vi "email.vi"(1 "Body":string="[No Body]", 2 "Enable":bool) -> ()   [LabVIEW 2011]
panel:
  out "error out":errorcluster
  in  "CC (Carbon Copy Recipient - Optional)":string
  in  "Attachment - Optional":path
  in  "Port":i32=587
  in  "Enable SSL":bool=TRUE
  in  "GMAIL Account Password":string="joblhzitaafwukgr"
  in  "GMAIL Account User ID":string="hvac.labview"
  in  "Outgoing Mail Server (SMTP)":string="smtp.gmail.com"
  in  "Subject":string="Automatic Email: HVAC Project"
  in  "Recipient's Name":string="HVAC Member"
  in  "Recipient's Email":string="mani.amoozadeh2@gmail.com"
  in  "Sender's Name":string="hvac.labview"
  in  "Sender's Email":string="hvac.labview@gmail.com"
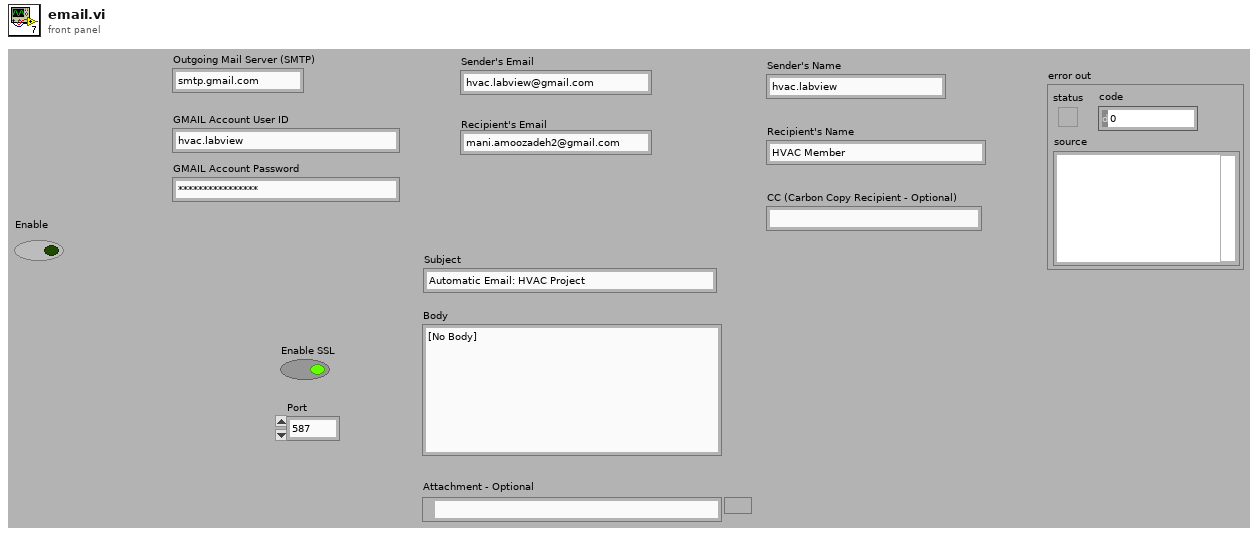
[diagram p1: front panel]
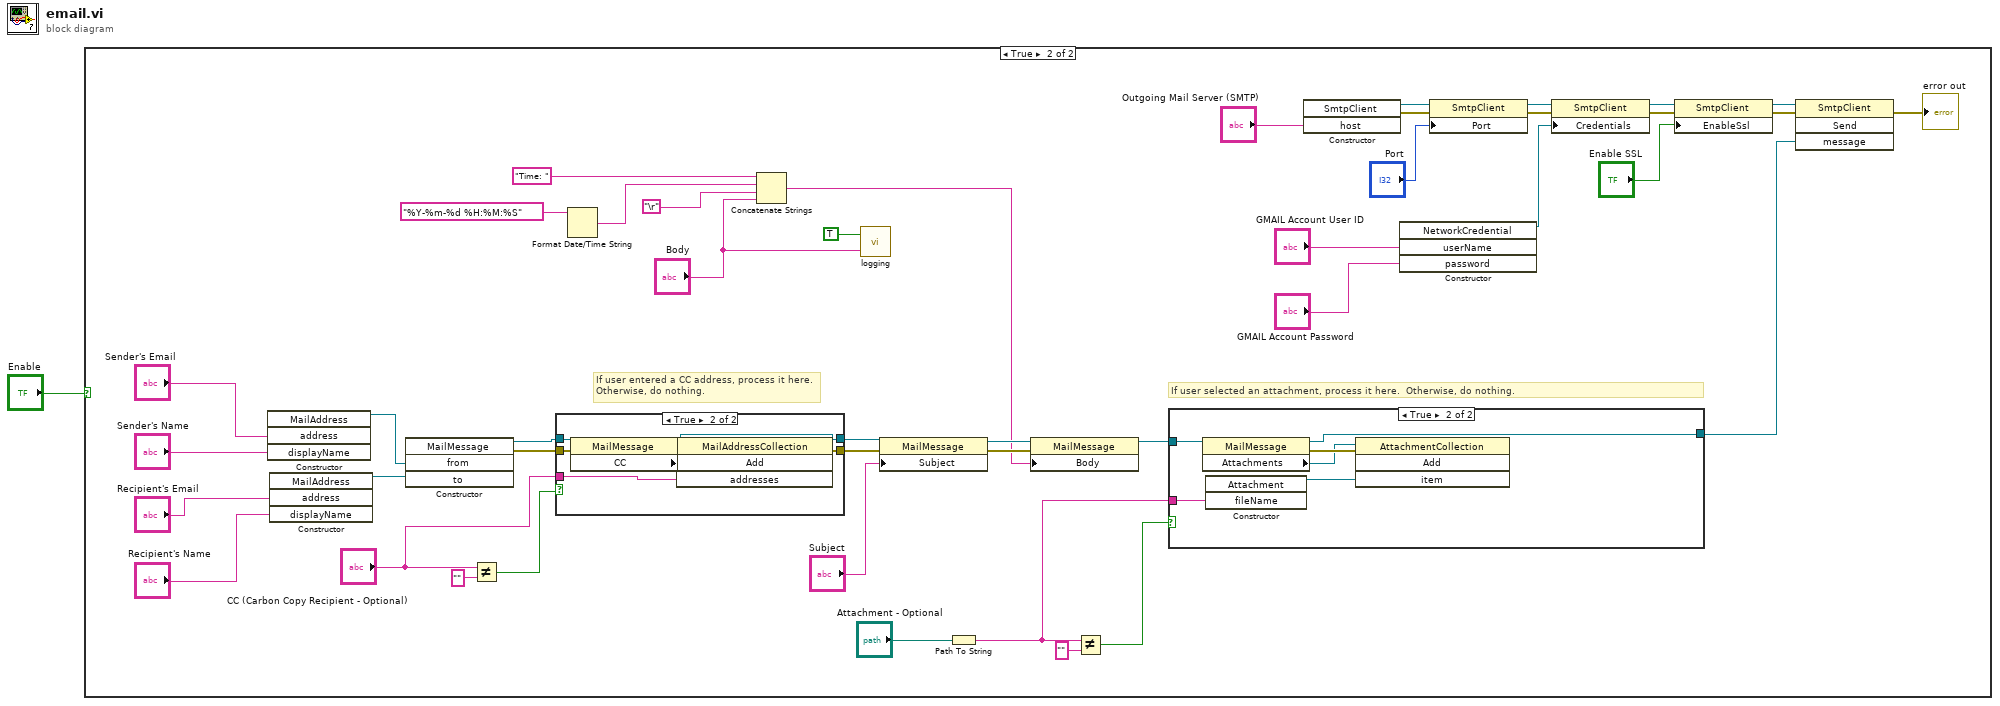
[diagram p0: block diagram]
diagram:
  n1 = case shown="True" "Enable" {
    frame False {
    }
    frame True {
      # "If user selected an attachment, process it here.  Otherwise, do nothing."
      # "If user entered a CC address, process it here.\nOtherwise, do nothing."
      n2 = constructor class="MailAddress"("address"="Sender's Email", "displayName"="Sender's Name") -> (reference out=w44:refnum<k24>)  [unwired: 3 in, 4 out]
      n3 = constructor class="MailAddress"("address"="Recipient's Email", "displayName"="Recipient's Name") -> (reference out=w45:refnum<k24>)  [unwired: 3 in, 4 out]
      n4 = constructor class="MailMessage"("from"=w44, "to"=w45) -> (reference out=w13:refnum<k24>, error out=w12:errorcluster)  [unwired: 3 in, 3 out]
      n5 = Not Equal?(x="CC (Carbon Copy Recipient - Optional)", y="") -> (x != y?=w15:bool)
      n6 = case shown="True" w15 {
        tunnel: "CC (Carbon Copy Recipient - Optional)" -> [_ w52]
        tunnel: w13 -> [w47 w51]
        tunnel: w12 -> [w46 w50]
        tunnel: [w47 w49] -> w11
        tunnel: [w46 w48] -> w10
        frame False {
        }
        frame True {
          n7 = property class="MailMessage"(reference=w51, error in=w50) -> (reference out=w49:refnum<k24>, error out=w54:errorcluster, "CC"=w53:refnum<k24>)
          n8 = invoke class="MailAddressCollection" method="Add"(reference=w53, error in=w54, "addresses"=w52) -> (error out=w48:errorcluster)  [unwired: 1 in, 3 out]
        }
      }
      n9 = Format Date/Time String(time format string (%c)="%Y-%m-%d %H:%M:%S") -> (date/time string=w5:string)  [unwired: 2 in]
      n10 = Concatenate Strings("Time: ", w5, "\r", "Body") -> (w3:string)
      n11 = call "logging.vi"("data"="Body", "Boolean"=TRUE) -> ()  [unwired: 1 in]
      n12 = property class="MailMessage"(reference=w11, error in=w10, "Subject"="Subject") -> (reference out=w36:refnum<k24>, error out=w43:errorcluster)
      n13 = Path To String(path="Attachment - Optional") -> (string=w17:string)
      n14 = property class="MailMessage"(reference=w36, error in=w43, "Body"=w3) -> (reference out=w22:refnum<k24>)  [unwired: 1 out]
      n15 = Not Equal?(x=w17, y="") -> (x != y?=w18:bool)
      n16 = case shown="True" w18 {
        tunnel: w22 -> [w55 w58]
        tunnel: [w55 w57] -> w21
        tunnel: w17 -> [_ w56]
        frame False {
        }
        frame True {
          n17 = property class="MailMessage"(reference=w58) -> (reference out=w57:refnum<k24>, error out=w61:errorcluster, "Attachments"=w59:refnum<k24>)  [unwired: 1 in]
          n18 = constructor class="Attachment"("fileName"=w56) -> (reference out=w60:refnum<k24>)  [unwired: 3 in, 3 out]
          n19 = invoke class="AttachmentCollection" method="Add"(reference=w59, error in=w61, "item"=w60) -> ()  [unwired: 1 in, 4 out]
        }
      }
      n20 = constructor class="SmtpClient"("host"="Outgoing Mail Server (SMTP)") -> (reference out=w30:refnum<k24>, error out=w26:errorcluster)  [unwired: 3 in, 2 out]
      n21 = constructor class="NetworkCredential"("userName"="GMAIL Account User ID", "password"="GMAIL Account Password") -> (reference out=w31:refnum<k24>)  [unwired: 3 in, 4 out]
      n22 = property class="SmtpClient"(reference=w30, error in=w26, "Port"="Port") -> (reference out=w29:refnum<k24>, error out=w25:errorcluster)
      n23 = property class="SmtpClient"(reference=w29, error in=w25, "Credentials"=w31) -> (reference out=w28:refnum<k24>, error out=w24:errorcluster)
      n24 = property class="SmtpClient"(reference=w28, error in=w24, "EnableSsl"="Enable SSL") -> (reference out=w27:refnum<k24>, error out=w23:errorcluster)
      n25 = invoke class="SmtpClient" method="Send"(reference=w27, error in=w23, "message"=w21) -> (error out=→"error out":errorcluster)  [unwired: 1 in, 3 out]
    }
  }
